vi "Set piezo um.vi"(0 "Piezo handle":i32, 5 "X pos (um)":dbl min=0.0 max=100.0, 7 "Y pos (um)":dbl min=0.0 max=100.0, 9 "Z pos (um)":dbl min=0.0 max=100.0, 11 "Piezo error in":errorcluster) -> (4 "Piezo handle out":i32, 15 "Piezo error out":errorcluster)   [LabVIEW 2017]
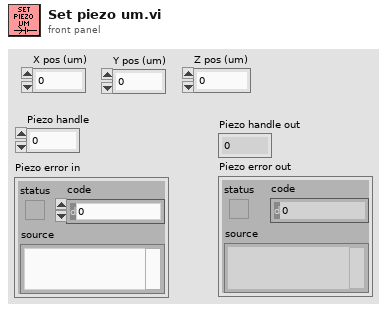
[diagram p1: front panel]
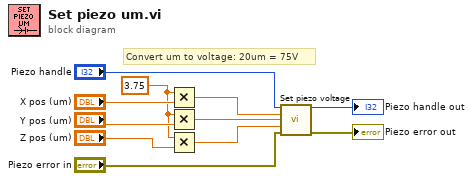
[diagram p0: block diagram]
diagram:
  w1 = 3.75 ("x")
  # "Convert um to voltage: 20um = 75V"
  n1 = Multiply(x=w1, y="X pos (um)") -> (x*y=w2:dbl)
  n2 = Multiply(x=w1, y="Y pos (um)") -> (x*y=w3:dbl)
  n3 = Multiply(x=w1, y="Z pos (um)") -> (x*y=w4:dbl)
  n4 = call "Set piezo voltage.vi"("Piezo handle"="Piezo handle", "X Voltage"=w2, "Y Voltage"=w3, "Z Voltage"=w4, "Piezo error in"="Piezo error in") -> ("Piezo handle out"=→"Piezo handle out":i32, "Piezo error out"=→"Piezo error out":errorcluster)  [unwired: 9 in]
